vi "PowerSlideInit.vi"(8 "PowerSlideReduction":dbl, 9 "PowerSlideTurnThreshold":dbl, 10 "PowerSlideRatio":bool) -> ()   [LabVIEW 2014, in "PowerSlide.lvlib"]
uses:
  PowerSlide.lvlib
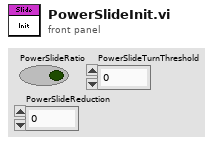
[diagram p1: front panel]
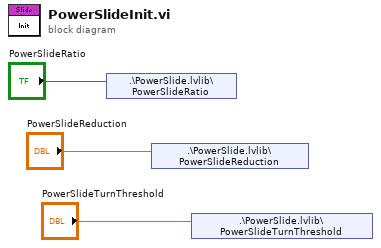
[diagram p0: block diagram]
diagram:
  n1 = shared-variable ".\\PowerSlide.lvlib\\PowerSlideRatio"("PowerSlideRatio") -> ()  [unwired: 1 in, 1 out]
  n2 = shared-variable ".\\PowerSlide.lvlib\\PowerSlideReduction"("PowerSlideReduction") -> ()  [unwired: 1 in, 1 out]
  n3 = shared-variable ".\\PowerSlide.lvlib\\PowerSlideTurnThreshold"("PowerSlideTurnThreshold") -> ()  [unwired: 1 in, 1 out]
